vi "Read Pulse Configuration.vi"(8 "error in (no error)":errorcluster, 11 "DAQmx DAQmx Digitizer in":refnum<class "DAQmx Digitizer.lvclass">) -> (0 "error out":errorcluster, 2 "Configuration":T1={"Post-trigger delay"=0.01, "Post-trigger duration"=0.1, "Rate"=1000000.0, "Ranges"=[10.0], "Re-name channels"=[], "Active channels"="0:1", "External clock"=FALSE} {"Rate" format="%#_8pHz"; "Post-trigger duration" format="%#_6ps"; "Post-trigger delay" format="%#_6ps"; "Ranges" format="%#_6pV"}, 3 "DAQmx DAQmx Digitizer in":refnum<class "DAQmx Digitizer.lvclass">)   [LabVIEW 2021, in "DAQmx Digitizer.lvclass"]
uses:
  DAQmx Digitizer.lvclass
  C:/GitHub/NHMFL_Core/Libraries/Instruments/Instrument Driver/Instrument Driver.lvclass
  Instruments/Pulse Driver/Pusle Driver Configuration.ctl
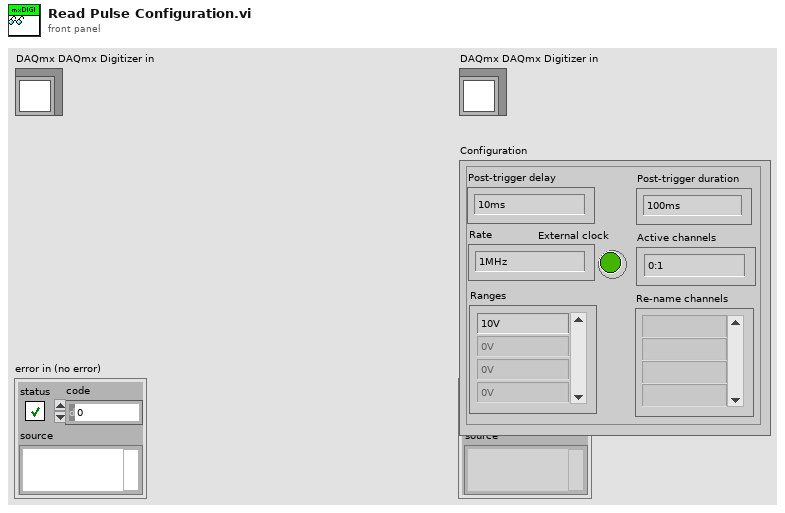
[diagram p1: front panel]
types:
  T1 = typedef "Pusle Driver Configuration.ctl" = cluster{"Post-trigger delay":dbl, "Post-trigger duration":dbl, "Rate":dbl, "Ranges":dbl[], "Re-name channels":string[], "Active channels":string, "External clock":bool}
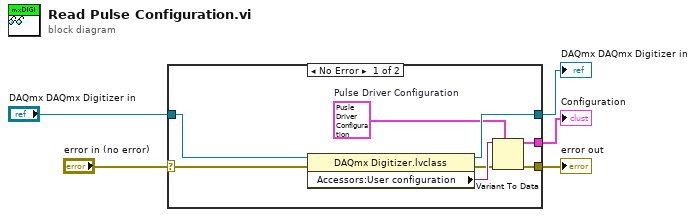
[diagram p0: block diagram]
diagram:
  n1 = case shown="No Error" "error in (no error)" {
    selector: "error in (no error)" -> [w6 w14]
    tunnel: [w8 w14] -> w4
    tunnel: [w12 w15] -> w2
    tunnel: "DAQmx DAQmx Digitizer in" -> [w13 w15]
    tunnel: [w9 _] -> w1
    frame No Error {
      w11 = T1 {"Post-trigger delay"=0.01, "Post-trigger duration"=0.1, "Rate"=1000000.0, "Ranges"=[10.0], "Re-name channels"=[], "Active channels"="0:1", "External clock"=FALSE}  # Pulse Driver Configuration
      n2 = property class="DAQmx Digitizer.lvclass"(reference=w13, error in=w6) -> (reference out=w12:refnum<class "DAQmx Digitizer.lvclass">, error out=w7:errorcluster, "Accessors:User configuration"=w10:variant)
      n3 = Variant To Data(error in=w7, type=w11, Variant=w10) -> (data=w9:T1, error out=w8:errorcluster)
    }
    frame Error {
    }
  }
  "error out" <- w4
  "DAQmx DAQmx Digitizer in" <- w2
  "Configuration" <- w1
